vi "Calibration_Save.vi"(0 "Img1":T3, 1 "Data":T1={"L16 Linear Actuator"="", "XE 1000 Pump"="", "Camera1"="", "Camera2"="", "Camera1_IMG"=refnum, "Camera2_IMG"=refnum, "Img_Capt"=FALSE, "Actuator"=FALSE, "Pump"=FALSE, "Cam 1"=FALSE, "Cam 2"=FALSE, "Empty_Refill"=FALSE, "Crop"=FALSE, "Light intensity"=0, "Exposure Time"=0.0, "Sample Name"="", "Operator"="", "Calibration 1"=path "", "Calibration 2"=path "", "Framerate"=0, "Timeout Sample"=0, "Collection date"="", "Sample size threshold"=1, "Empty start"=1, "Command"="MRJ", "Calibration Image 1"=refnum, "Calibration Image 2"=refnum, "Original Image 1"=refnum, "Original Image 2"=refnum, "Processing Image 1"=refnum, "Processing Image 2"=refnum, "Object Image 1"=refnum, "Object Image 2"=refnum, "Station"="", "Species Name"="", "Other Notes"="", "Aperture"=enum."Item 0", "Image Process Queue Size"=500, "Image Save Queue Size"=500, "Overload threshold"=500, "Max Framerate"=100, "Blue Plane Image"=refnum, "Subtract Image"=refnum, "Binary Image 1"=refnum, "ROI mask allocation"=refnum, "Rectangle 1"={"Left"=0, "Top"=0, "Right"=0, "Bottom"=0, "Rotation"=0.0}, "Rectangle 2"={"Left"=0, "Top"=0, "Right"=0, "Bottom"=0, "Rotation"=0.0}, "Binary Image 2"=refnum, "Detection Region %"=0.0, "Cam 1 queue"=refnum, "Cam 2 queue"=refnum, "Detect image 1"=refnum, "Detect image 2"=refnum, "Detect 1"=path "C:/Users/au540322/Desktop/IHS_Project/images/Debris/Debris_0/Debris_0_2019_06_01-23-32-49-686.PNG", "Detect 2"=path "C:/Users/au540322/Desktop/IHS_Project/images/Debris/Debris_0/Debris_0_2019_06_01-23-32-49-686.PNG", "Max large object threshold"=0, "Open(T)/Close(F)"=FALSE, "Cam 1 - save queue"=refnum, "Cam 2 - save queue"=refnum, "Img_Capt Begin"=FALSE, "Image Save 1"=refnum, "Image Save 2"=refnum, "Dispense Speed"=100, "Flush Size"=100} {"Flush Size" min=1; "Dispense Speed" min=1; "Rectangle 2"."Rotation" format="%.2f"; "Rectangle 2"."Left" scale=0.0..1024.0; "Rectangle 2"."Right" scale=0.0..1024.0; "Rectangle 1"."Rotation" format="%.2f"; "Rectangle 1"."Left" scale=0.0..1024.0; "Rectangle 1"."Right" scale=0.0..1024.0; "Max Framerate" min=1; "Overload threshold" min=1; "Image Save Queue Size" min=1; "Image Process Queue Size" min=1; "Empty start" min=1; "Sample size threshold" min=1; "Framerate" min=1; "Light intensity" scale=0.0..100.0}, 5 "Img2":T3, 9 "Dtct":bool, 11 "Crop?":bool) -> (4 "Cal1":path, 6 "Cal2":path, 8 "Data out":T1={"L16 Linear Actuator"="", "XE 1000 Pump"="", "Camera1"="", "Camera2"="", "Camera1_IMG"=refnum, "Camera2_IMG"=refnum, "Img_Capt"=FALSE, "Actuator"=FALSE, "Pump"=FALSE, "Cam 1"=FALSE, "Cam 2"=FALSE, "Empty_Refill"=FALSE, "Crop"=FALSE, "Light intensity"=0, "Exposure Time"=0.0, "Sample Name"="", "Operator"="", "Calibration 1"=path "", "Calibration 2"=path "", "Framerate"=0, "Timeout Sample"=0, "Collection date"="", "Sample size threshold"=1, "Empty start"=1, "Command"="MRJ", "Calibration Image 1"=refnum, "Calibration Image 2"=refnum, "Original Image 1"=refnum, "Original Image 2"=refnum, "Processing Image 1"=refnum, "Processing Image 2"=refnum, "Object Image 1"=refnum, "Object Image 2"=refnum, "Station"="", "Species Name"="", "Other Notes"="", "Aperture"=enum."Item 0", "Image Process Queue Size"=500, "Image Save Queue Size"=500, "Overload threshold"=500, "Max Framerate"=100, "Blue Plane Image"=refnum, "Subtract Image"=refnum, "Binary Image 1"=refnum, "ROI mask allocation"=refnum, "Rectangle 1"={"Left"=0, "Top"=0, "Right"=0, "Bottom"=0, "Rotation"=0.0}, "Rectangle 2"={"Left"=0, "Top"=0, "Right"=0, "Bottom"=0, "Rotation"=0.0}, "Binary Image 2"=refnum, "Detection Region %"=0.0, "Cam 1 queue"=refnum, "Cam 2 queue"=refnum, "Detect image 1"=refnum, "Detect image 2"=refnum, "Detect 1"=path "C:/Users/au540322/Desktop/IHS_Project/images/Debris/Debris_0/Debris_0_2019_06_01-23-32-49-686.PNG", "Detect 2"=path "C:/Users/au540322/Desktop/IHS_Project/images/Debris/Debris_0/Debris_0_2019_06_01-23-32-49-686.PNG", "Max large object threshold"=0, "Open(T)/Close(F)"=FALSE, "Cam 1 - save queue"=refnum, "Cam 2 - save queue"=refnum, "Img_Capt Begin"=FALSE, "Image Save 1"=refnum, "Image Save 2"=refnum, "Dispense Speed"=100, "Flush Size"=100} {"Flush Size" min=1; "Dispense Speed" min=1; "Rectangle 2"."Rotation" format="%.2f"; "Rectangle 2"."Left" scale=0.0..1024.0; "Rectangle 2"."Right" scale=0.0..1024.0; "Rectangle 1"."Rotation" format="%.2f"; "Rectangle 1"."Left" scale=0.0..1024.0; "Rectangle 1"."Right" scale=0.0..1024.0; "Max Framerate" min=1; "Overload threshold" min=1; "Image Save Queue Size" min=1; "Image Process Queue Size" min=1; "Empty start" min=1; "Sample size threshold" min=1; "Framerate" min=1; "Light intensity" scale=0.0..100.0}, 10 "Img1 out":T3, 15 "Img2 out":T3)   [LabVIEW 2019]
uses:
  controls/Data.ctl
  <vilib>/userdefined/High Color/IMAQdx.ctl
  <vilib>/vision/Image Controls.llb/IMAQ Image.ctl
panel:
  out "error out 2":errorcluster
  out "error out":errorcluster
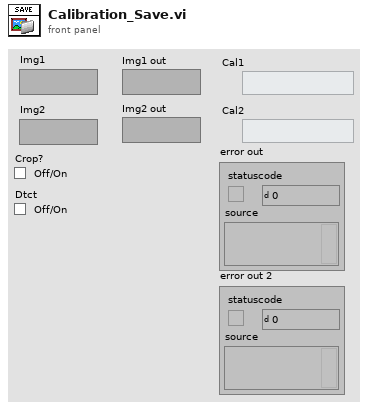
[diagram p1: front panel]
types:
  T1 = typedef "Data.ctl" = cluster{"L16 Linear Actuator":refnum<visa-resource-name>, "XE 1000 Pump":refnum<visa-resource-name>, "Camera1":T2, "Camera2":T2, "Camera1_IMG":T3, "Camera2_IMG":T3, "Img_Capt":bool, "Actuator":bool, "Pump":bool, "Cam 1":bool, "Cam 2":bool, "Empty_Refill":bool, "Crop":bool, "Light intensity":i32, "Exposure Time":dbl, "Sample Name":string, "Operator":string, "Calibration 1":path, "Calibration 2":path, "Framerate":i32, "Timeout Sample":i32, "Collection date":string, "Sample size threshold":i32, "Empty start":u32, "Command":string, "Calibration Image 1":T3, "Calibration Image 2":T3, "Original Image 1":T3, "Original Image 2":T3, "Processing Image 1":T3, "Processing Image 2":T3, "Object Image 1":T3, "Object Image 2":T3, "Station":string, "Species Name":string, "Other Notes":string, "Aperture":enum32{"Item 0", "Item 1", "Item 2", "Item 3"}, "Image Process Queue Size":i32, "Image Save Queue Size":i32, "Overload threshold":i32, "Max Framerate":i32, "Blue Plane Image":T3, "Subtract Image":T3, "Binary Image 1":T3, "ROI mask allocation":T3, "Rectangle 1":T4, "Rectangle 2":T4, "Binary Image 2":T3, "Detection Region %":dbl, "Cam 1 queue":refnum<queue>, "Cam 2 queue":refnum<queue>, "Detect image 1":T3, "Detect image 2":T3, "Detect 1":path, "Detect 2":path, "Max large object threshold":i32, "Open(T)/Close(F)":bool, "Cam 1 - save queue":refnum<queue>, "Cam 2 - save queue":refnum<queue>, "Img_Capt Begin":bool, "Image Save 1":T3, "Image Save 2":T3, "Dispense Speed":i32, "Flush Size":i32}
  T2 = typedef "IMAQdx.ctl" = refnum<k21>
  T3 = typedef "IMAQ Image.ctl" = refnum<image>
  T4 = typedef "IMAQ Rectangle" = cluster{"Left":i32, "Top":i32, "Right":i32, "Bottom":i32, "Rotation":dbl}
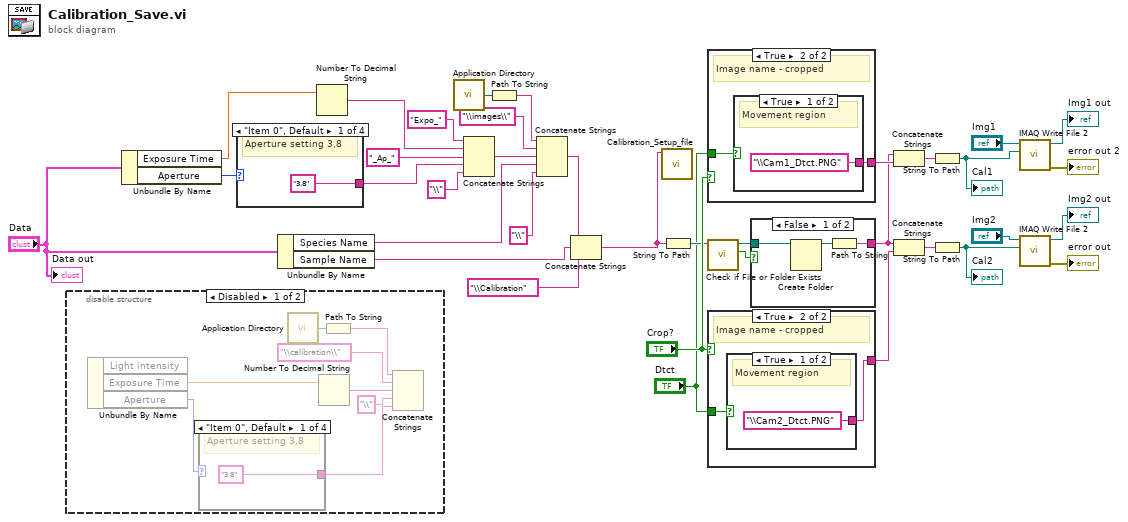
[diagram p0: block diagram]
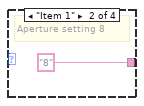
[diagram p2: hidden frame]
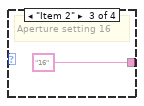
[diagram p3: hidden frame]
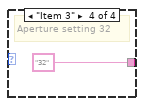
[diagram p4: hidden frame]
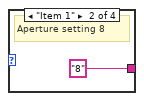
[diagram p6: hidden frame]
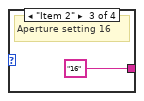
[diagram p7: hidden frame]
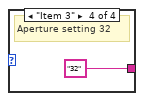
[diagram p8: hidden frame]
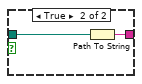
[diagram p9: hidden frame]
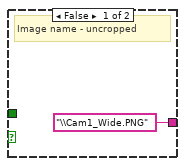
[diagram p10: hidden frame]
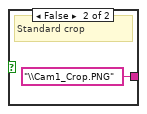
[diagram p11: hidden frame]
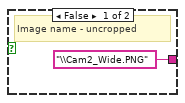
[diagram p12: hidden frame]
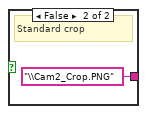
[diagram p13: hidden frame]
diagram:
  n1 = disable-structure shown="Disabled" {
    frame Disabled {
      n2 = Unbundle By Name() -> ("Exposure Time"=w43:dbl, "Aperture"=w37:enum32{"Item 0", "Item 1", "Item 2", "Item 3"})  [unwired: 1 in, 1 out]
      n3 = case shown="\"Item 0\", Default" w37 {
        tunnel: ["3.8" "8" "16" "32"] -> w38
        frame "Item 0", Default {
          # "Aperture setting 3,8"
        }
        frame "Item 1" {
          # "Aperture setting 8"
        }
        frame "Item 2" {
          # "Aperture setting 16"
        }
        frame "Item 3" {
          # "Aperture setting 32"
        }
      }
      n4 = call <vilib>:"Application Directory.vi"() -> ("Application Directory"=w40:path)
      n5 = Number To Decimal String(number=w43) -> (decimal integer string=w42:string)  [unwired: 1 in]
      n6 = Path To String(path=w40) -> (string=w39:string)
      n7 = Concatenate Strings(w39, "\\calibration\\" ("string"), w42, "\\" ("string"), w38) -> ()  [unwired: 1 out]
    }
    frame Enabled {
    }
  }
  n8 = Unbundle By Name("Data") -> ("Exposure Time"=w11:dbl, "Aperture"=w8:enum32{"Item 0", "Item 1", "Item 2", "Item 3"})
  n9 = case shown="\"Item 0\", Default" w8 {
    tunnel: ["3.8" "8" "16" "32"] -> w6
    frame "Item 0", Default {
      # "Aperture setting 3,8"
    }
    frame "Item 1" {
      # "Aperture setting 8"
    }
    frame "Item 2" {
      # "Aperture setting 16"
    }
    frame "Item 3" {
      # "Aperture setting 32"
    }
  }
  n10 = Unbundle By Name("Data") -> ("Species Name"=w15:string, "Sample Name"=w13:string)
  n11 = Number To Decimal String(number=w11) -> (decimal integer string=w7:string)  [unwired: 1 in]
  n12 = call <vilib>:"Application Directory.vi"() -> ("Application Directory"=w16:path)
  n13 = Concatenate Strings("Expo_" ("string"), w7, "_Ap_" ("string"), w6, "\\" ("string")) -> (w4:string)
  n14 = Path To String(path=w16) -> (string=w17:string)
  n15 = Concatenate Strings(w17, "\\images\\" ("string"), w4, w15, "\\" ("string")) -> (w14:string)
  n16 = Concatenate Strings(w14, w13, "\\Calibration" ("string")) -> (w2:string)
  n17 = call "Calibration_Setup_file.vi"("Path"=w2) -> ()  [unwired: 11 in]
  n18 = String To Path(string=w2) -> (path=w21:path)
  n19 = case shown="True" "Crop?" {
    tunnel: ["\\Cam1_Wide.PNG" ("string") w55] -> w35
    tunnel: "Dtct" -> [_ w54]
    frame False {
      # "Image name - uncropped"
    }
    frame True {
      # "Image name - cropped"
      n20 = case shown="True" w54 {
        tunnel: ["\\Cam1_Dtct.PNG" ("string") "\\Cam1_Crop.PNG" ("string")] -> w55
        frame True {
          # "Movement region"
        }
        frame False {
          # "Standard crop"
        }
      }
    }
  }
  n21 = call <vilib>:"Check if File or Folder Exists.vi"("path"=w21) -> ("file or folder exists?"=w23:bool, "dup path"=w22:path)  [unwired: 8 in, 1 out]
  n22 = case shown="True" "Crop?" {
    tunnel: ["\\Cam2_Wide.PNG" ("string") w60] -> w36
    tunnel: "Dtct" -> [_ w59]
    frame False {
      # "Image name - uncropped"
    }
    frame True {
      # "Image name - cropped"
      n23 = case shown="True" w59 {
        tunnel: ["\\Cam2_Dtct.PNG" ("string") "\\Cam2_Crop.PNG" ("string")] -> w60
        frame True {
          # "Movement region"
        }
        frame False {
          # "Standard crop"
        }
      }
    }
  }
  n24 = case shown="False" w23 {
    tunnel: w22 -> [w65 w67]
    tunnel: [w63 w66] -> w20
    frame False {
      n25 = Create Folder(path (use dialog)=w65) -> (created path=w64:path)  [unwired: 2 in, 2 out]
      n26 = Path To String(path=w64) -> (string=w63:string)
    }
    frame True {
      n27 = Path To String(path=w67) -> (string=w66:string)
    }
  }
  n28 = Concatenate Strings(w20, w35) -> (w34:string)
  n29 = Concatenate Strings(w20, w36) -> (w33:string)
  n30 = String To Path(string=w34) -> (path=w26:path)
  "Cal1" <- w26
  n31 = String To Path(string=w33) -> (path=w32:path)
  "Cal2" <- w32
  n32 = call-poly "IMAQ Write File 2"("File Path"=w26, "Image"="Img1") -> ("error out"=→"error out 2":errorcluster, "Image Out (duplicate)"=→"Img1 out":T3)  [unwired: 8 in]
  n33 = call-poly "IMAQ Write File 2"("File Path"=w32, "Image"="Img2") -> ("error out"=→"error out":errorcluster, "Image Out (duplicate)"=→"Img2 out":T3)  [unwired: 8 in]
  "Data out" <- "Data"
